vi "DestroyWindow.vi"(8 "No Error":errorcluster, 11 "Window [SDL_Window*]":i64) -> (0 "error out":errorcluster)   [LabVIEW 2024, in "SDL3.lvlib" / "Video.lvlib"]
doc: "<B>Summary</B>\nDestroy a window."
uses:
  Video.lvlib
  Lib/SDL3-32.dll
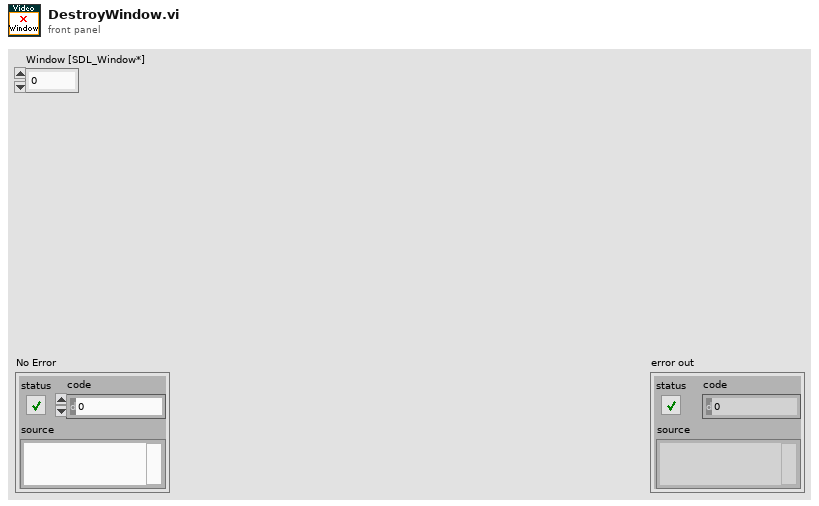
[diagram p1: front panel]
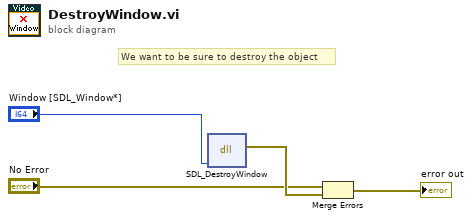
[diagram p0: block diagram]
diagram:
  # "We want to be sure to destroy the object"
  n1 = dll-call lib="C:/Users/Thomas/Documents/Projects/LV-SDL3/Lib/SDL3-*.*" fn="SDL_DestroyWindow"("window"="Window [SDL_Window*]") -> (error out=w4:errorcluster)  [unwired: 5 in, 1 out]
  n2 = Merge Errors("No Error", w4) -> (→"error out":errorcluster)
